vi "Write LargeFileObjectAvailable.vi"(8 "error in (no error)":errorcluster, 10 "LargeFileObjectAvailable":refnum<user-event>, 11 "ElectrometerController in":refnum<class "ElectrometerController.lvclass">) -> (0 "error out":errorcluster, 3 "ElectrometerController out":refnum<class "ElectrometerController.lvclass">)   [LabVIEW 2016, in "ElectrometerController.lvclass"]
uses:
  ElectrometerController.lvclass
  ts_sallv_calibrationelectrometer/DataTypes/logevent_LargeFileObjectAvailable.ctl
  ElectrometerController.lvclass/ElectrometerController.ctl
  ts_sallv_calibrationelectrometer/SALLV_calibrationElectrometer.lvlib
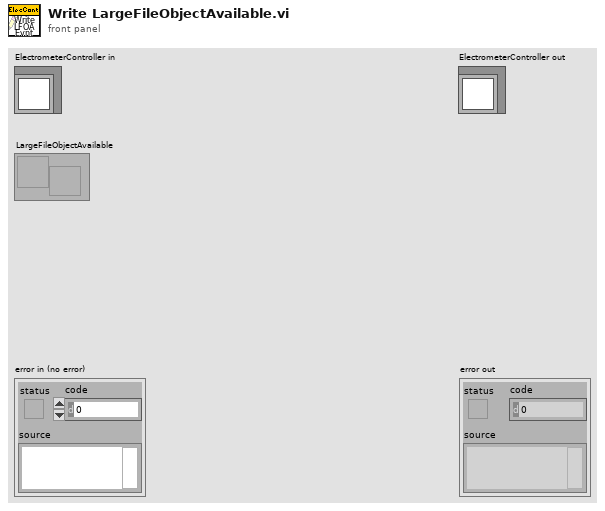
[diagram p1: front panel]
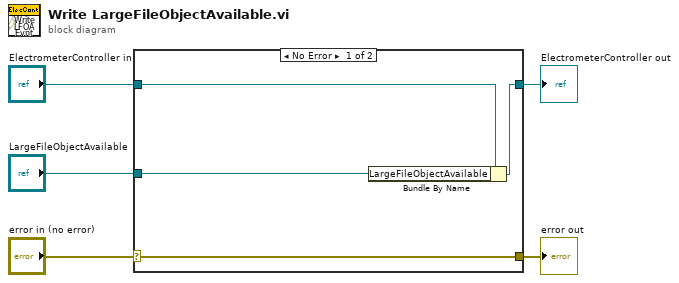
[diagram p0: block diagram]
diagram:
  n1 = case shown="No Error" "error in (no error)" {
    selector: "error in (no error)" -> [w9 w10]
    tunnel: [w9 w10] -> w4
    tunnel: [w7 w11] -> w2
    tunnel: "ElectrometerController in" -> [w8 w11]
    tunnel: "LargeFileObjectAvailable" -> [w6 _]
    frame No Error {
      n2 = Bundle By Name(cluster=w8, "LargeFileObjectAvailable"=w6) -> (w7:refnum<class "ElectrometerController.lvclass">)
    }
    frame Error {
    }
  }
  "error out" <- w4
  "ElectrometerController out" <- w2
